vi "Get Tree Data Definitions.vi"(8 "Error In":errorcluster, 11 "Tree Manager":T1) -> (0 "Error Out":errorcluster, 1 "Tree Data Defs":refnum<class "Tree Data.lvclass">[](array[class]), 3 "Tree Manager":T1)   [LabVIEW 2020, in "NI_VIAnCFGDataStructure.lvlib" / "Tree.lvclass"]
doc: "Get the definitions of Tree Data classes used to recognize, flatten and unflatten XML and LV Tree Control."
uses:
  <vilib>/addons/analyzer/VIAnCFGDataStructure/Tree Manager/Tree.lvclass
  <vilib>/addons/analyzer/VIAnCFGDataStructure/Tree Manager/Typedefs/Session Handle.ctl
  <vilib>/addons/analyzer/VIAnCFGDataStructure/Tree Data/Tree Data.lvclass
  <vilib>/addons/analyzer/VIAnCFGDataStructure/Tree Manager/Tree.lvclass/Tree.ctl
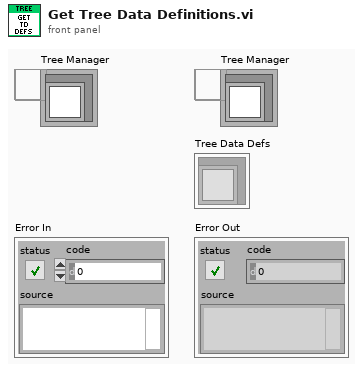
[diagram p1: front panel]
types:
  T1 = typedef "NI_VIAnCFGDataStructure.lvlib/Tree.lvclass/Session Handle.ctl" = refnum<data-value>
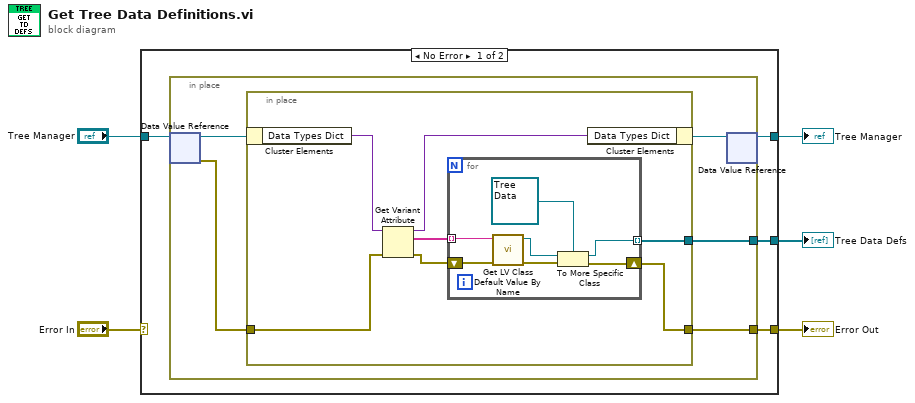
[diagram p0: block diagram]
diagram:
  n1 = case shown="No Error" "Error In" {
    selector: "Error In" -> [_ w29]
    tunnel: "Tree Manager" -> [w9 w30]
    tunnel: [w8 w30] -> w4
    tunnel: [w7 w29] -> w2
    tunnel: [w6 _] -> w1
    frame No Error {
      n2 = in-place {
        in-place-border: [w13] -> w7
        in-place-border: [w10] -> w6
        n3 = in-place-dvr #1(w9) -> (w14:refnum<class "Tree.lvclass">, w11:errorcluster)
        n4 = in-place {
          in-place-border: [w15] -> w13
          in-place-border: w11 -> [w18]
          in-place-border: [w19] -> w10
          n5 = in-place-cluster #2(w14) -> ("Data Types Dict"=w21:variant)
          n6 = Get Variant Attribute(Variant=w21, error in=w18) -> (duplicate Variant=w20:variant, names=w17:string[], error out=w16:errorcluster)  [unwired: 2 in, 1 out]
          n7 = for {
            tunnel: [w25] -> w19 mode=indexing
            tunnel: w17 -> [w24] mode=indexing
            shift-right: [w22] -> w15
            shift-left: w16 -> [w23]
            n8 = call <vilib>:"Get LV Class Default Value By Name.vi"("error in (no error)"=w23, "class name"=w24) -> ("error out"=w28:errorcluster, "object"=w27:refnum<class>)  [unwired: 8 in]
            n9 = To More Specific Class(target class=refnum<class "Tree Data.lvclass"> refnum ("Tree Data.lvclass"), reference=w27, error in=w28) -> (specific class reference=w25:refnum<class "Tree Data.lvclass">, error out=w22:errorcluster)
          }
          n10 = in-place-cluster #2("Data Types Dict"=w20) -> (w12:refnum<class "Tree.lvclass">)
        }
        n11 = in-place-dvr #1(w12) -> (w8:T1)  [unwired: 1 out]
      }
    }
    frame Error {
    }
  }
  "Tree Manager" <- w4
  "Error Out" <- w2
  "Tree Data Defs" <- w1
